vi "Tranrate.vi"(6 "timeout (ms)(10000)":i32=10000, 7 "DeepL authKey":string, 8 "error in (no error)":errorcluster caption="エラー入力 (エラーなし)", 10 "TargetLang":T2, 11 "Input text":string) -> (0 "エラー出力":errorcluster, 3 "translations":T1(array[cluster]))   [LabVIEW 2015, in "lv-deepl-api.lvlib"]
uses:
  lv-deepl-api.lvlib
  TargetLang.ctl
  <vilib>/httpClient/POSTBuffer.vi
  <vilib>/httpClient/LabVIEWHTTPClient.lvlib
panel:
  out "headers":string
  out "body":string
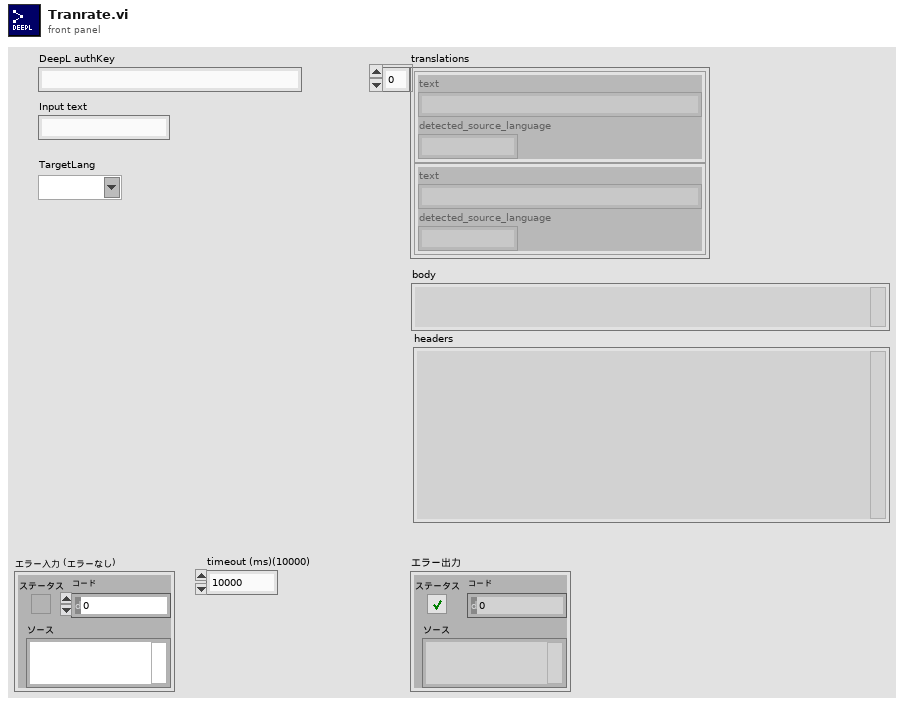
[diagram p1: front panel]
types:
  T1 = cluster{"detected_source_language":string, "text":string}[]
  T2 = typedef "TargetLang.ctl" = string
  T3 = typedef "LabVIEWHTTPClient.lvlib/ClientHandle.ctl" = refnum<k1>
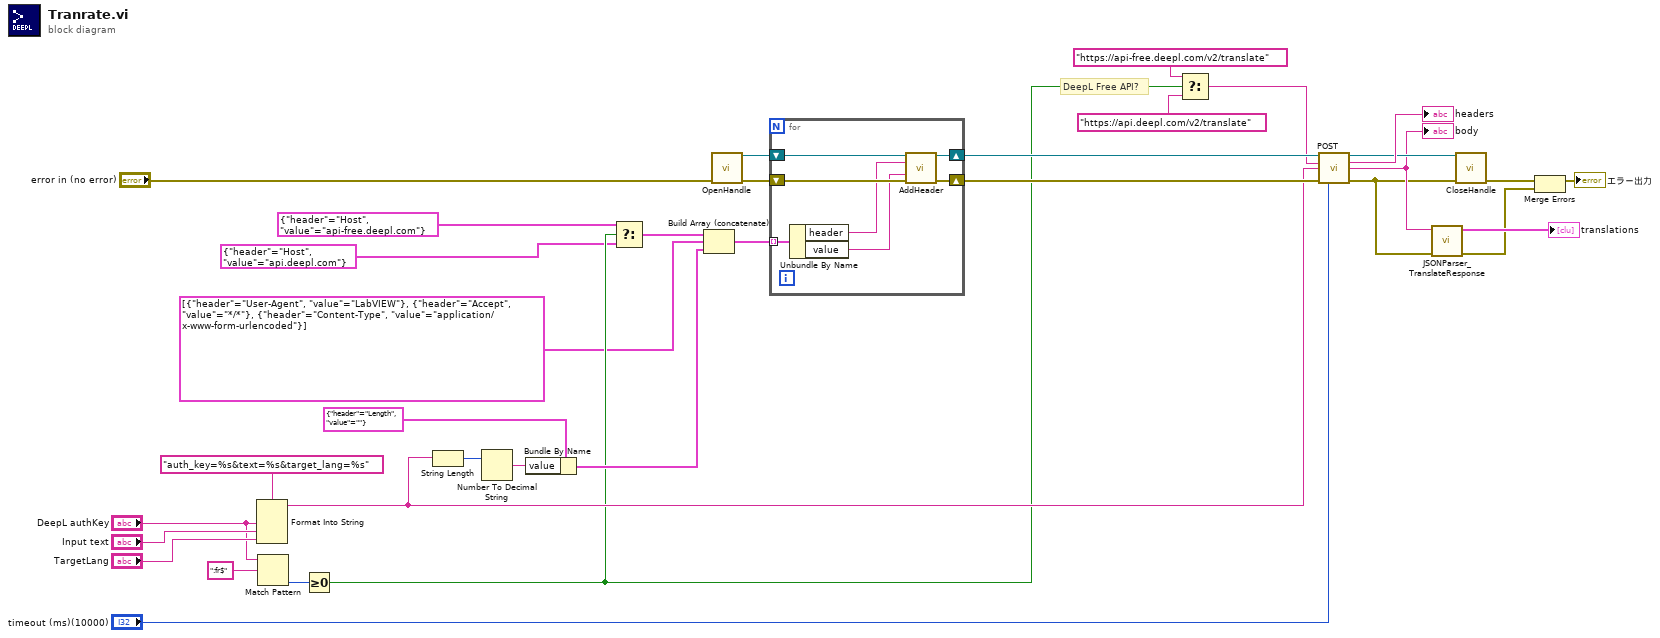
[diagram p0: block diagram]
diagram:
  # "DeepL Free API?"
  n1 = Format Into String(format string="auth_key=%s&text=%s&target_lang=%s" ("url"), "DeepL authKey", "Input text", "TargetLang") -> (resulting string=w22:string)  [unwired: 2 in, 1 out]
  n2 = Match Pattern(string="DeepL authKey", regular expression=":fr$" ("正規表現")) -> (offset past match=w11:i32)  [unwired: 1 in, 3 out]
  n3 = Greater Or Equal To 0?(x=w11) -> (x >= 0?=w7:bool)
  n4 = String Length(string=w22) -> (length=w25:i32)
  n5 = Number To Decimal String(number=w25) -> (decimal integer string=w24:string)  [unwired: 1 in]
  n6 = Bundle By Name(cluster=cluster{"header":string, "value":string} {"header"="Length", "value"=""} ("Cluster"), "value"=w24) -> (w27:cluster{"header":string, "value":string})
  n7 = Select(t=cluster{"header":string, "value":string} {"header"="Host", "value"="api-free.deepl.com"} ("Cluster"), s=w7, f=cluster{"header":string, "value":string} {"header"="Host", "value"="api.deepl.com"} ("Cluster")) -> (s? t:f=w4:cluster{"header":string, "value":string})
  n8 = Build Array (concatenate)(w4, cluster{"header":string, "value":string}[] [{"header"="User-Agent", "value"="LabVIEW"}, {"header"="Accept", "value"="*/*"}, {"header"="Content-Type", "value"="application/x-www-form-urlencoded"}], w27) -> (w26:cluster{"header":string, "value":string}[])
  n9 = call <vilib>:"OpenHandle.vi"("error in (no error)"="error in (no error)") -> ("client handle out"=w34:T3, "error out"=w33:errorcluster)  [unwired: 13 in]
  n10 = for {
    shift-right: [w39] -> w32
    shift-left: w34 -> [w41]
    shift-right: [w38] -> w31
    shift-left: w33 -> [w40]
    tunnel: w26 -> [w37] mode=indexing
    n11 = Unbundle By Name(w37) -> ("header"=w36:string, "value"=w35:string)
    n12 = call <vilib>:"AddHeader.vi"("client handle"=w41, "header"=w36, "value"=w35, "error in (no error)"=w40) -> ("client handle out"=w39:T3, "error out"=w38:errorcluster)  [unwired: 10 in]
  }
  n13 = Select(t="https://api-free.deepl.com/v2/translate" ("url"), s=w7, f="https://api.deepl.com/v2/translate" ("url")) -> (s? t:f=w9:string)
  n14 = call-poly <vilib>:"POST.vi"("client handle"=w32, "url"=w9, "buffer"=w22, "error in (no error)"=w31, "timeout (10000)"="timeout (ms)(10000)") -> ("client handle out"=w29:T3, "headers"=→"headers":string, "body"=w19:string, "error out"=w2:errorcluster)  [unwired: 7 in]
  "body" <- w19
  n15 = call "JSONParser_TranslateResponse.vi"("error in (no error)"=w2, "JSON Text"=w19) -> ("error out"=w16:errorcluster, "translations"=→"translations":T1)  [unwired: 8 in]
  n16 = call <vilib>:"CloseHandle.vi"("client handle"=w29, "error in (no error)"=w2) -> ("error out"=w17:errorcluster)  [unwired: 13 in]
  n17 = Merge Errors(w17, w16) -> (→"エラー出力":errorcluster)
